vi "Easy2Acquire.IComponent.Enable.vi"(0 "Motion.Select":T1=[{"Component"="line.human.pelvis;type.input.motion.rot;device.noraxon.imu.3;", "Collect"=TRUE}, {"Component"="line.human.pelvis.magnetometer.enable;type.command;device.noraxon.imu.3;", "Collect"=FALSE}, {"Component"="line.human.pelvis.magnetometer.disable;type.command;device.noraxon.imu.3;", "Collect"=FALSE}, {"Component"="line.human.pelvis;type.input.motion.accel;device.noraxon.imu.3;", "Collect"=FALSE}, {"Component"="line.magnetometer.reset;device.noraxon.imu.3;type.command;", "Collect"=FALSE}, {"Component"="line.magnetometer.enable;device.noraxon.imu.3;type.command;", "Collect"=FALSE}, {"Component"="line.magnetometer.disable;device.noraxon.imu.3;type.command;", "Collect"=FALSE}], 1 "Digital.Select":T1, 3 "AnalogFreq":dbl, 4 "Analog.Select":T1, 5 "error in (no error)":errorcluster, 6 "ComponentCount":i32, 7 "IDeviceIn":refnum<k7>) -> (15 "AnalogInput":refnum<k7>[](array[refnum]), 17 "DigitalInput":refnum<k7>[](array[refnum]), 18 "MotionInput":refnum<k7>[](array[refnum]), 19 "error out":errorcluster)   [LabVIEW 2017]
uses:
  MM-MotionSelect-CTRL.ctl
panel:
  in  "Easy2AcquireCom.IMotionInput":refnum<k7>
  in  "Easy2AcquireCom.IDigitalInput":refnum<k7>
  in  "Easy2AcquireCom.IAnalogInput":refnum<k7>
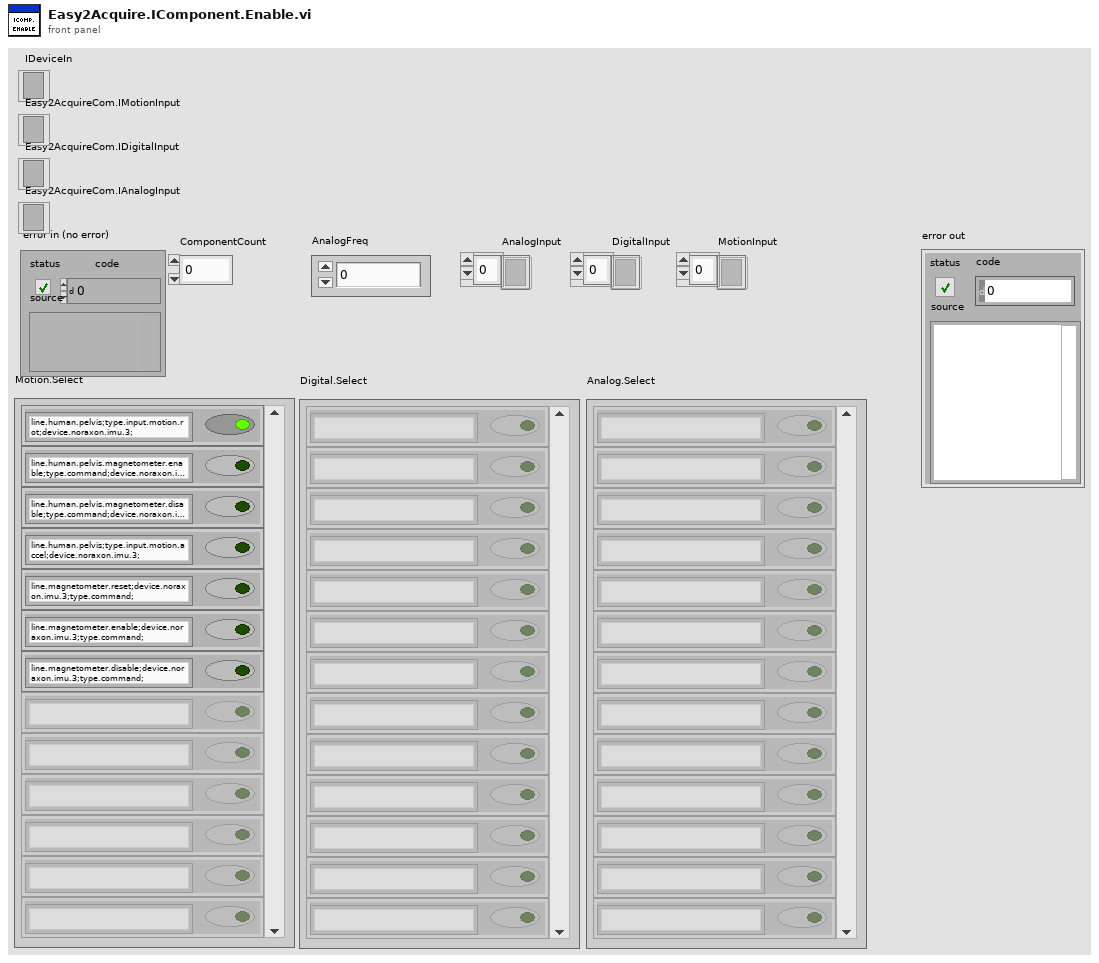
[diagram p1: front panel]
types:
  T1 = typedef "MM-MotionSelect-CTRL.ctl" = cluster{"Component":string, "Collect":bool}[]
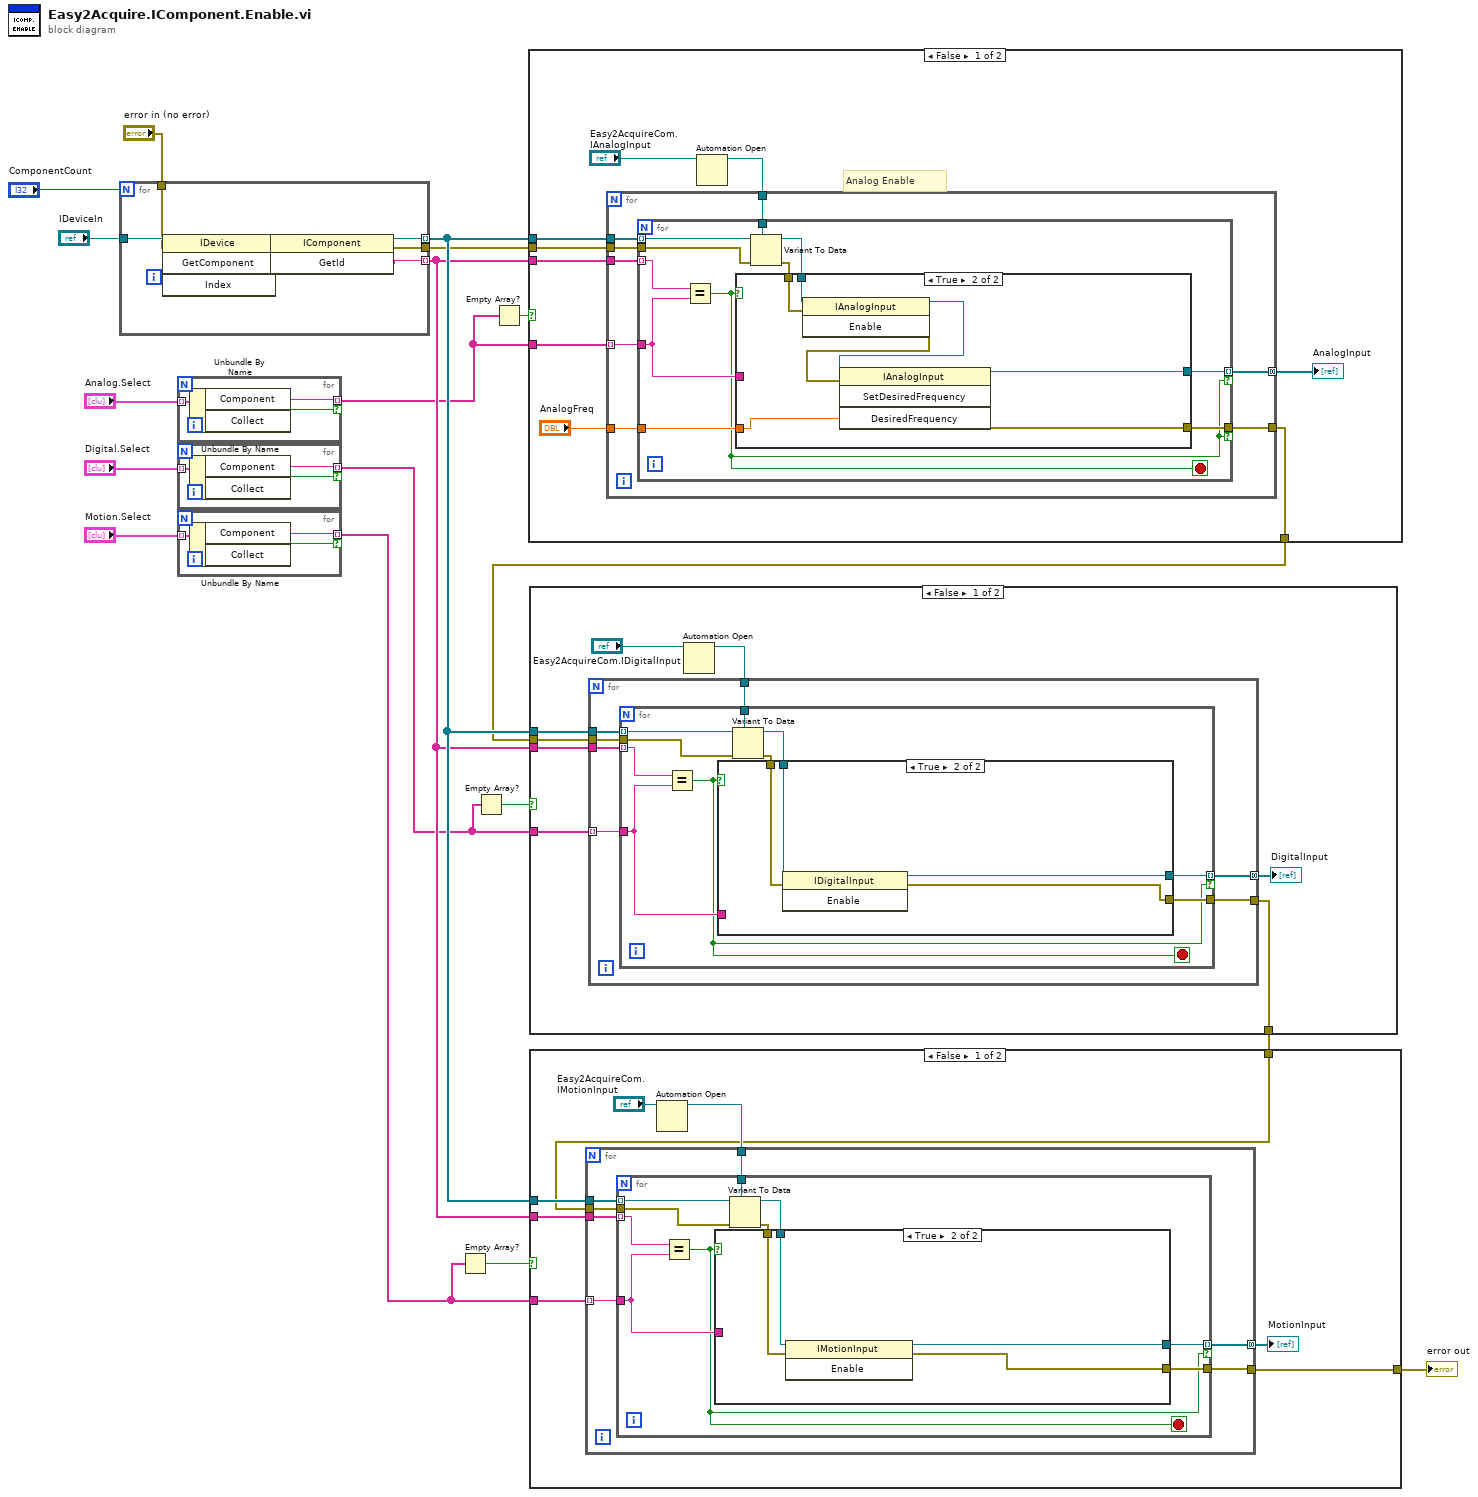
[diagram p0: block diagram]
diagram:
  n1 = for {
    N: "ComponentCount" -> [_]
    tunnel: [w23] -> w12 mode=indexing
    tunnel: "IDeviceIn" -> [w22]
    tunnel: [w21] -> w13 mode=indexing
    tunnel: [w20] -> w11
    tunnel: "error in (no error)" -> [w19]
    i -> [w24]
    n2 = invoke class="IDevice" method="GetComponent"(reference=w22, error in=w19, "Index"=w24) -> (error out=w25:errorcluster, "GetComponent"=w26:refnum<k7>)  [unwired: 1 in, 2 out]
    n3 = invoke class="IComponent" method="GetId"(reference=w26, error in=w25) -> (reference out=w21:refnum<k7>, error out=w20:errorcluster, "GetId"=w23:string)  [unwired: 1 in]
  }
  n4 = for {
    tunnel: "Analog.Select" -> [w29] mode=indexing
    tunnel: [w28] -> w7 mode=indexing if=w27
    n5 = Unbundle By Name(w29) -> ("Component"=w28:string, "Collect"=w27:bool)
  }
  n6 = for {
    tunnel: "Digital.Select" -> [w32] mode=indexing
    tunnel: [w31] -> w4 mode=indexing if=w30
    n7 = Unbundle By Name(w32) -> ("Component"=w31:string, "Collect"=w30:bool)
  }
  n8 = for {
    tunnel: "Motion.Select" -> [w35] mode=indexing
    tunnel: [w34] -> w1 mode=indexing if=w33
    n9 = Unbundle By Name(w35) -> ("Component"=w34:string, "Collect"=w33:bool)
  }
  n10 = Empty Array?(array=w1) -> (empty?=w2:bool)
  n11 = Empty Array?(array=w4) -> (empty?=w5:bool)
  n12 = Empty Array?(array=w7) -> (empty?=w6:bool)
  n13 = case shown="False" w6 {
    tunnel: w7 -> [w43 _]
    tunnel: w13 -> [w40 _]
    tunnel: w12 -> [w39 _]
    tunnel: w11 -> [w38 w72]
    tunnel: [w37 w72] -> w9
    frame False {
      # "Analog Enable"
      n14 = Automation Open(Automation Refnum="Easy2AcquireCom.IAnalogInput") -> (Automation Refnum=w42:refnum<k7>)  [unwired: 3 in, 1 out]
      n15 = for {
        tunnel: w43 -> [w51] mode=indexing
        tunnel: w39 -> [w52]
        tunnel: w40 -> [w50]
        tunnel: w42 -> [w49]
        tunnel: w38 -> [w48]
        tunnel: [w47] -> w36 mode=concatenating
        tunnel: [w46] -> w37
        tunnel: "AnalogFreq" -> [w45]
        n16 = for {
          tunnel: w52 -> [w63] mode=indexing
          tunnel: w51 -> [w56]
          tunnel: w50 -> [w62] mode=indexing
          tunnel: w49 -> [w61]
          tunnel: w48 -> [w58]
          tunnel: [w57] -> w47 mode=indexing if=w53
          tunnel: [w55] -> w46 if=w53
          tunnel: w45 -> [w54]
          stop <- w53 stop-if-true
          n17 = Equal?(x=w63, y=w56) -> (x = y?=w53:bool)
          n18 = Variant To Data(error in=w58, type=w61, Variant=w62) -> (data=w60:refnum<k7>, error out=w59:errorcluster)
          n19 = case shown="True" w53 {
            tunnel: w60 -> [_ w71]
            tunnel: w59 -> [w64 w70]
            tunnel: [_ w65] -> w57
            tunnel: w56 -> [_ _]
            tunnel: [w64 w66] -> w55
            tunnel: w54 -> [_ w67]
            frame False {
            }
            frame True {
              n20 = invoke class="IAnalogInput" method="Enable"(reference=w71, error in=w70) -> (reference out=w68:refnum<k7>, error out=w69:errorcluster)  [unwired: 1 in, 1 out]
              n21 = invoke class="IAnalogInput" method="SetDesiredFrequency"(reference=w68, error in=w69, "DesiredFrequency"=w67) -> (reference out=w65:refnum<k7>, error out=w66:errorcluster)  [unwired: 1 in, 2 out]
            }
          }
        }
      }
      "AnalogInput" <- w36
    }
    frame True {
    }
  }
  n22 = case shown="False" w5 {
    tunnel: w4 -> [w78 _]
    tunnel: w13 -> [w76 _]
    tunnel: w12 -> [w75 _]
    tunnel: [w74 w103] -> w10
    tunnel: w9 -> [w73 w103]
    frame False {
      n23 = Automation Open(Automation Refnum="Easy2AcquireCom.IDigitalInput") -> (Automation Refnum=w79:refnum<k7>)  [unwired: 3 in, 1 out]
      n24 = for {
        tunnel: w78 -> [w86] mode=indexing
        tunnel: w75 -> [w87]
        tunnel: w76 -> [w85]
        tunnel: w79 -> [w84]
        tunnel: w73 -> [w83]
        tunnel: [w82] -> w77 mode=concatenating
        tunnel: [w81] -> w74
        n25 = for {
          tunnel: w87 -> [w97] mode=indexing
          tunnel: w86 -> [w90]
          tunnel: w85 -> [w96] mode=indexing
          tunnel: w84 -> [w95]
          tunnel: w83 -> [w92]
          tunnel: [w91] -> w82 mode=indexing if=w88
          tunnel: [w89] -> w81
          stop <- w88 stop-if-true
          n26 = Equal?(x=w97, y=w90) -> (x = y?=w88:bool)
          n27 = Variant To Data(error in=w92, type=w95, Variant=w96) -> (data=w94:refnum<k7>, error out=w93:errorcluster)
          n28 = case shown="True" w88 {
            tunnel: w94 -> [_ w102]
            tunnel: w93 -> [w98 w101]
            tunnel: [_ w100] -> w91
            tunnel: w90 -> [_ _]
            tunnel: [w98 w99] -> w89
            frame False {
            }
            frame True {
              n29 = invoke class="IDigitalInput" method="Enable"(reference=w102, error in=w101) -> (reference out=w100:refnum<k7>, error out=w99:errorcluster)  [unwired: 1 in, 1 out]
            }
          }
        }
      }
      "DigitalInput" <- w77
    }
    frame True {
    }
  }
  n30 = case shown="False" w2 {
    tunnel: w13 -> [w111 _]
    tunnel: w12 -> [w110 _]
    tunnel: w1 -> [w109 _]
    tunnel: w10 -> [w105 w134]
    tunnel: [w104 w134] -> w3
    frame False {
      n31 = Automation Open(Automation Refnum="Easy2AcquireCom.IMotionInput") -> (Automation Refnum=w108:refnum<k7>)  [unwired: 3 in, 1 out]
      n32 = for {
        tunnel: w109 -> [w117] mode=indexing
        tunnel: w110 -> [w118]
        tunnel: w111 -> [w116]
        tunnel: w105 -> [w115]
        tunnel: [w114] -> w106 mode=concatenating
        tunnel: [w113] -> w104
        tunnel: w108 -> [w112]
        n33 = for {
          tunnel: w118 -> [w128] mode=indexing
          tunnel: w117 -> [w122]
          tunnel: w116 -> [w127] mode=indexing
          tunnel: w115 -> [w124]
          tunnel: [w123] -> w114 mode=indexing if=w120
          tunnel: [w121] -> w113
          tunnel: w112 -> [w119]
          stop <- w120 stop-if-true
          n34 = Equal?(x=w128, y=w122) -> (x = y?=w120:bool)
          n35 = Variant To Data(error in=w124, type=w119, Variant=w127) -> (data=w126:refnum<k7>, error out=w125:errorcluster)
          n36 = case shown="True" w120 {
            tunnel: w126 -> [_ w132]
            tunnel: w125 -> [w129 w133]
            tunnel: [_ w131] -> w123
            tunnel: w122 -> [_ _]
            tunnel: [w129 w130] -> w121
            frame False {
            }
            frame True {
              n37 = invoke class="IMotionInput" method="Enable"(reference=w132, error in=w133) -> (reference out=w131:refnum<k7>, error out=w130:errorcluster)  [unwired: 1 in, 1 out]
            }
          }
        }
      }
      "MotionInput" <- w106
    }
    frame True {
    }
  }
  "error out" <- w3
